vi "Notifier-with-memory-graphTabs.vi"(8 "error in":errorcluster, 10 "Timeout [ms]":i32, 11 "Display-tab":refnum<notifier>) -> (0 "error IO":errorcluster, 2 "Notification":T1)   [LabVIEW 2013, in "CameraVision.lvlib" / "CV-UI.lvclass"]
doc: "Polymorphic type of Notifier-with-memory vi.\n\nAccepts a notifier reference for an instance of the type-defined control 'Displays'.\nThe vi listens for 'Timeout' miliseconds for a new message on the notifier.\nIf no message arrives or arrived before calling the vi, the last received message is returned.\n\nThe default message is 'Last image'."
uses:
  CV-UI.lvclass
  Display-selector.ctl
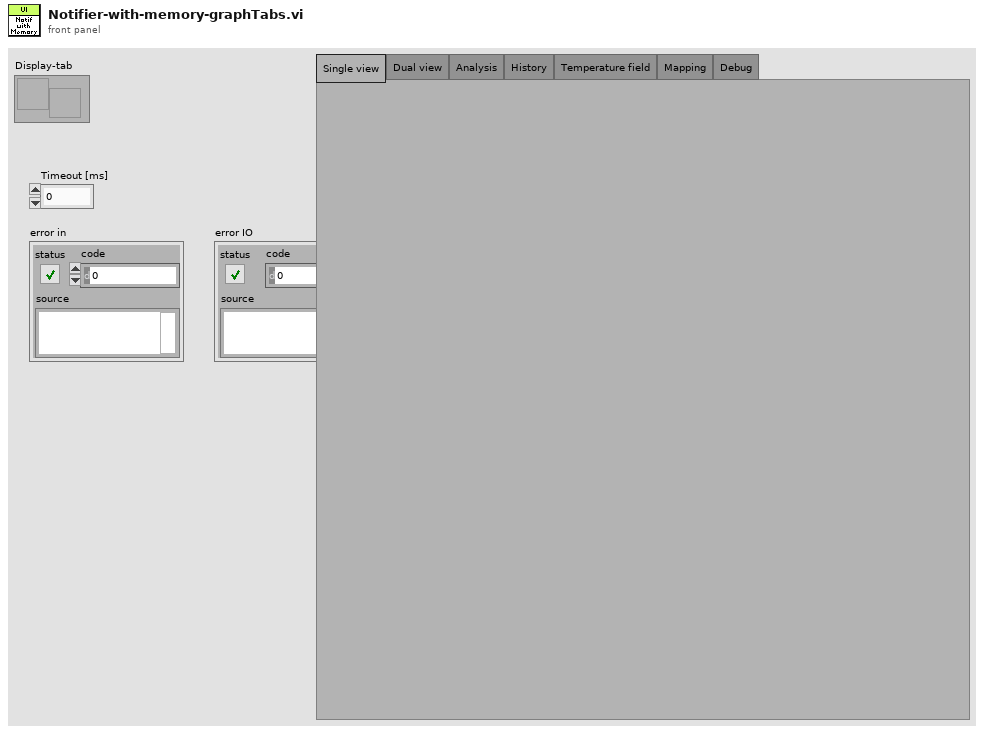
[diagram p1: front panel]
types:
  T1 = typedef "CameraVision.lvlib/CV-UI.lvclass/Display-selector.ctl" = enum32{"Single view", "Dual view", "Analysis", "History", "Temperature field", "Mapping", "Debug"}
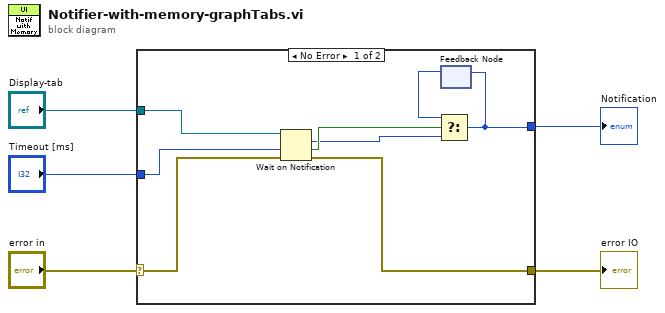
[diagram p0: block diagram]
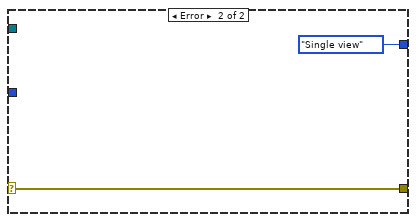
[diagram p2: hidden frame]
diagram:
  n1 = case shown="No Error" "error in" {
    selector: "error in" -> [w6 w14]
    tunnel: [w13 w14] -> w5
    tunnel: "Timeout [ms]" -> [w12 _]
    tunnel: "Display-tab" -> [w8 _]
    tunnel: [w7 Display-selector."Single view" ("Displays")] -> w2
    frame No Error {
      n2 = Wait on Notification(notifier=w8, timeout in ms (-1)=w12, error in (no error)=w6) -> (notification=w10:T1, timed out?=w11:bool, error out=w13:errorcluster)  [unwired: 1 in, 1 out]
      n3 = feedback #1() -> (w9:T1)  [unwired: 1 in]
      n4 = Select(t=w9, s=w11, f=w10) -> (s? t:f=w7:T1)
      n5 = feedback-in #1(w7) -> ()
    }
    frame Error {
    }
  }
  "error IO" <- w5
  "Notification" <- w2
